vi "sendCommand.vi"(8 "error in (no error)":errorcluster, 10 "command":string, 11 "K2602 in":refnum<class "K2602.lvclass">) -> (0 "error out":errorcluster, 3 "K2602 out":refnum<class "K2602.lvclass">)   [LabVIEW 2011, in "Hardware.lvlib" / "Channels.lvlib" / "K2602.lvclass"]
uses:
  K2602.lvclass
  K2602.lvclass/K2602.ctl
  <instrlib>/Keithley 2600 Series/Keithley 2600 Series.lvlib
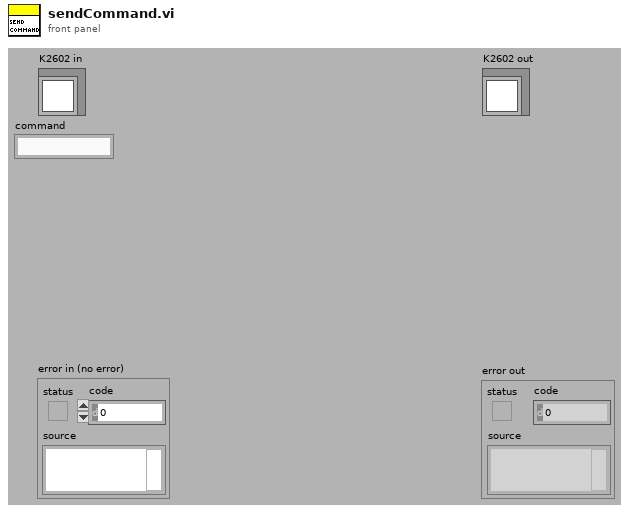
[diagram p1: front panel]
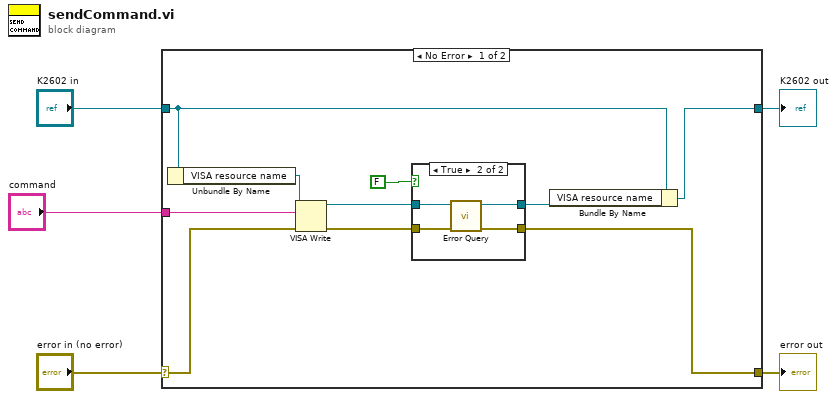
[diagram p0: block diagram]
diagram:
  n1 = case shown="No Error" "error in (no error)" {
    selector: "error in (no error)" -> [w13 w23]
    tunnel: [w12 w23] -> w4
    tunnel: [w7 w22] -> w2
    tunnel: "K2602 in" -> [w8 w22]
    tunnel: "command" -> [w11 _]
    frame No Error {
      n2 = Unbundle By Name(w8) -> ("VISA resource name"=w10:refnum<visa-resource-name>)
      n3 = VISA Write(VISA resource name=w10, write buffer=w11, error in (no error)=w13) -> (VISA resource name out=w15:refnum<visa-resource-name>, error out=w14:errorcluster)  [unwired: 1 out]
      n4 = case shown="True" FALSE {
        tunnel: w15 -> [w17 w21]
        tunnel: w14 -> [w16 w20]
        tunnel: [w17 w19] -> w6
        tunnel: [w16 w18] -> w12
        frame False {
        }
        frame True {
          n5 = call <instrlib>:"Error Query.vi"("error in (no error)"=w20, "VISA resource name"=w21) -> ("error out"=w18:errorcluster, "VISA resource name out"=w19:refnum<visa-resource-name>)  [unwired: 8 out]
        }
      }
      n6 = Bundle By Name(cluster=w8, "VISA resource name"=w6) -> (w7:refnum<class "K2602.lvclass">)
    }
    frame Error {
    }
  }
  "error out" <- w4
  "K2602 out" <- w2
